vi "hash_array_to_string_hash.vi"(8 "error in (no error)":errorcluster, 11 "message-digest":u8[](array[numeric])) -> (0 "error out":errorcluster, 3 "result string":string)   [LabVIEW 2015]
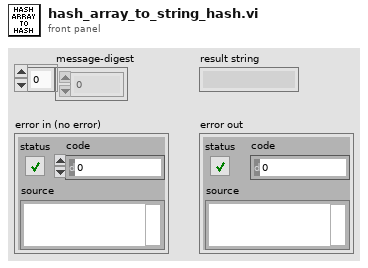
[diagram p1: front panel]
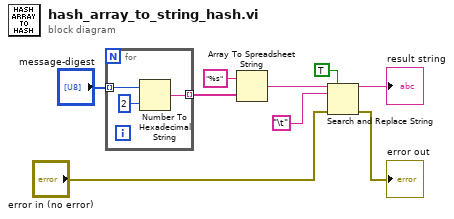
[diagram p0: block diagram]
diagram:
  n1 = for {
    tunnel: "message-digest" -> [w12] mode=indexing
    tunnel: [w11] -> w2 mode=indexing
    n2 = Number To Hexadecimal String(1:i16 2 ("width (-)"), 2:w12) -> (0:w11:string)
  }
  n3 = Array To Spreadsheet String(array=w2, 3:"%s" ("format string")) -> (spreadsheet string=w7:string)  [unwired: 1 in]
  n4 = Search and Replace String(replace all?=TRUE ("replace all? (F)"), input string=w7, search string="\t", error in="error in (no error)") -> (result string=→"result string":string, error out=→"error out":errorcluster)  [unwired: 4 in, 2 out]
